vi "fluigent_test.vi"() -> ()   [LabVIEW 2018]
uses:
  <userlib>/Fluigent/Fluigent MFCS/FluigentMFCS_Full.llb/_EZmfcsSN.ctl
  <userlib>/Fluigent/Fluigent MFCS/FluigentMFCS_Full.llb/MFCS_EZ Detect.vi
  <userlib>/Fluigent/Fluigent MFCS/FluigentMFCS_Full.llb/MFCS_EZ Initialization.vi
  <userlib>/Fluigent/Fluigent MFCS/FluigentMFCS_Full.llb/MFCS_EZ Write Channel Pressure.vi
  <userlib>/Fluigent/Fluigent MFCS/FluigentMFCS_Full.llb/MFCS_EZ Read Channel Pressure.vi
  <userlib>/Fluigent/Fluigent MFCS/FluigentMFCS_Full.llb/MFCS_EZ Close.vi
panel:
  out "[SN MFCS_EZ]":T1[](array[typedef])
  out "Numeric":dbl
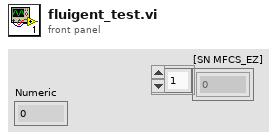
[diagram p1: front panel]
types:
  T1 = typedef "_EZmfcsSN.ctl" = u16
  T2 = typedef "_mfcs_EZ_handle.ctl" = u64
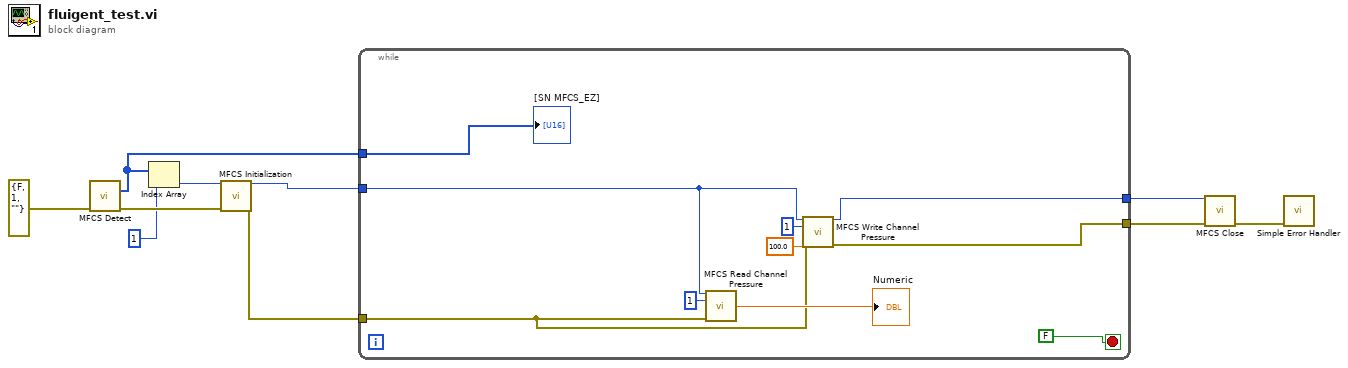
[diagram p0: block diagram]
diagram:
  n1 = call-poly <userlib>:"MFCS Detect.vi"("error in (no error)"=errorcluster {"status"=FALSE, "code"=1, "source"=""}) -> ("[SN MFCS_EZ]"=w2:T1[], "error out"=w9:errorcluster)  [unwired: 13 in]
  n2 = Index Array(array=w2, index=1) -> (element=w10:T1)
  n3 = call-poly <userlib>:"MFCS Initialization.vi"("SN MFCS_EZ"=w10, "error in (no error)"=w9) -> ("MFCS_EZ_out"=w7:T2, "error out"=w6:errorcluster)  [unwired: 10 in, 2 out]
  n4 = while {
    tunnel: w7 -> [w15]
    tunnel: w6 -> [w14]
    tunnel: [w13] -> w4
    tunnel: [w12] -> w3
    tunnel: w2 -> [w11]
    stop <- FALSE stop-if-true
    n5 = call-poly <userlib>:"MFCS Read Channel Pressure.vi"("MFCS_EZ"=w15, "Channel Number (default=1)"=u8 1, "error in (no error)"=w14) -> ("Pressure (mBar)"=→"Numeric":dbl)  [unwired: 9 in, 3 out]
    n6 = call-poly <userlib>:"MFCS Write Channel Pressure.vi"("MFCS_EZ"=w15, "Channel Number (default=1)"=u8 1, "Pressure (mBar)"=100.0, "error in (no error)"=w14) -> ("MFCS_EZ out"=w13:T2, "error out"=w12:errorcluster)  [unwired: 10 in]
    "[SN MFCS_EZ]" <- w11
  }
  n7 = call-poly <userlib>:"MFCS Close.vi"("MFCS_EZ"=w4, "error in (no error)"=w3) -> ("error out"=w5:errorcluster)  [unwired: 13 in]
  n8 = call <vilib>:"Simple Error Handler.vi"("error in (no error)"=w5) -> ()  [unwired: 4 in, 5 out]
